vi "Default Data.vi"(2 "Num Rows":i32, 3 "Aerotech_Soloist in":refnum<class "Aerotech_Soloist.lvclass">) -> (0 "Default Data":string[][](table)=[["CYCLE RESET", "Default", "0", "25"]], 1 "Aerotech_Soloist out":refnum<class "Aerotech_Soloist.lvclass">)   [LabVIEW 2013, in "Aerotech_Soloist.lvclass"]
doc: "Fill existing rows with 0's, unless specifically overridden."
uses:
  Aerotech_Soloist.lvclass
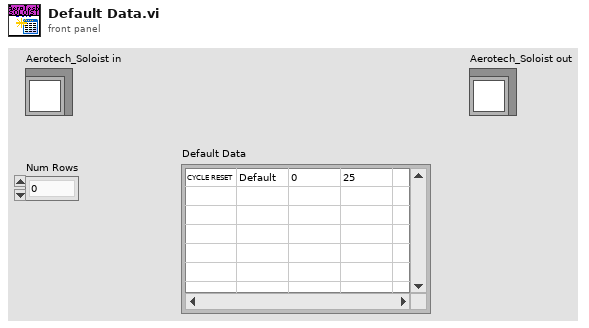
[diagram p1: front panel]
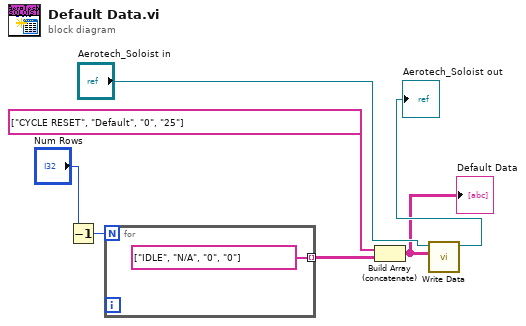
[diagram p0: block diagram]
diagram:
  n1 = Decrement(x="Num Rows") -> (x-1=w7:i32)
  n2 = for {
    N: w7 -> [_]
    tunnel: [string[] ["IDLE", "N/A", "0", "0"]] -> w6 mode=indexing
  }
  n3 = Build Array (concatenate)(string[] ["CYCLE RESET", "Default", "0", "25"], w6) -> (w2:string[][])
  "Default Data" <- w2
  n4 = call-dynamic "Write Data.vi"("Data"=w2, "Device in"="Aerotech_Soloist in") -> ("Device Out"=→"Aerotech_Soloist out":refnum<class "Aerotech_Soloist.lvclass">)  [unwired: 8 in, 1 out]
